vi "MPExxx_Auto_Seq_example.vi"() -> ()   [LabVIEW 2012]
doc: "This VI form enables the user to program the memory locations for auto sequencing mode and to intiate the auto sequencing mode.."
panel:
  out "error out":errorcluster
  in  "error in (no error)":errorcluster
  in  "?":enum32{"Sets Values", "Initiates Sequence"}(tab)
  in  "Memory Location":u8
  in  "Period":dbl format="%.2f"
  in  "OCP":dbl format="%.2f"
  in  "OVP":dbl format="%.2f"
  in  "Current":dbl format="%.2f"
  in  "Voltage":dbl format="%.2f"
  in  "Arm for Sequence":bool
  in  "Start":bool
  in  "VISA Resource Name":refnum<visa-resource-name>
  # "MAGNA-POWER"
  # "Electronics"
  # "Set Values for each memory location."
  # "ON"
  # "ON"
  # "OFF"
  # "OFF"
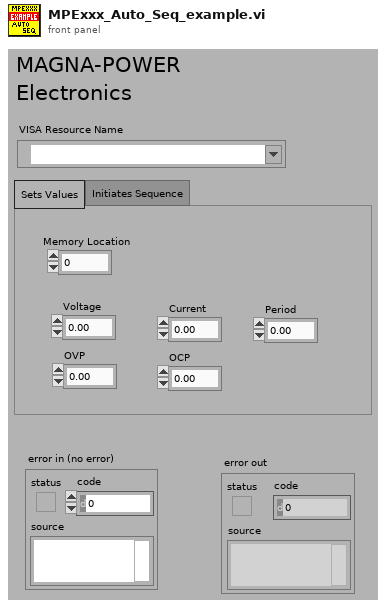
[diagram p1: front panel]
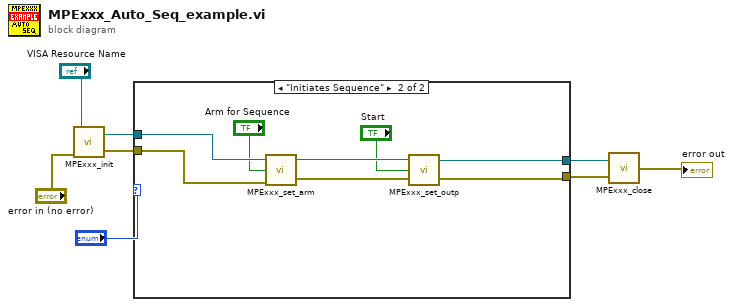
[diagram p0: block diagram]
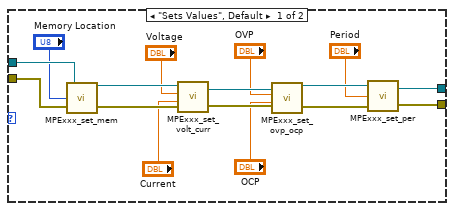
[diagram p2: hidden frame]
diagram:
  n1 = call "MPExxx_init.vi"("error in (no error)"="error in (no error)", "VISA session"="VISA Resource Name") -> ("error out"=w5:errorcluster, "dup VISA session"=w6:refnum<visa-resource-name>)  [unwired: 2 in]
  n2 = case shown="\"Initiates Sequence\"" "?" {
    tunnel: w6 -> [w24 w31]
    tunnel: w5 -> [w23 w32]
    tunnel: [w16 w27] -> w3
    tunnel: [w15 w28] -> w4
    frame "Sets Values", Default {
      n3 = call "MPExxx_set_mem.vi"("error in (no error)"=w23, "Set Mem"="Memory Location", "VISA session"=w24) -> ("error out"=w22:errorcluster, "dup VISA session"=w21:refnum<visa-resource-name>)
      n4 = call "MPExxx_set_volt_curr.vi"("error in (no error)"=w22, "Set Current"="Current", "Set Voltage"="Voltage", "VISA session"=w21) -> ("error out"=w20:errorcluster, "dup VISA session"=w19:refnum<visa-resource-name>)
      n5 = call "MPExxx_set_ovp_ocp.vi"("error in (no error)"=w20, "Set OCP"="OCP", "Set OVP"="OVP", "VISA session"=w19) -> ("error out"=w18:errorcluster, "dup VISA session"=w17:refnum<visa-resource-name>)
      n6 = call "MPExxx_set_per.vi"("error in (no error)"=w18, "Set Period"="Period", "VISA session"=w17) -> ("error out"=w15:errorcluster, "dup VISA session"=w16:refnum<visa-resource-name>)
    }
    frame "Initiates Sequence" {
      n7 = call "MPExxx_set_arm.vi"("error in (no error)"=w32, "ARM"="Arm for Sequence", "VISA session"=w31) -> ("error out"=w30:errorcluster, "dup VISA session"=w29:refnum<visa-resource-name>)
      n8 = call "MPExxx_set_outp.vi"("error in (no error)"=w30, "Output Control"="Start", "VISA session"=w29) -> ("error out"=w28:errorcluster, "dup VISA session"=w27:refnum<visa-resource-name>)
    }
  }
  n9 = call "MPExxx_close.vi"("error in (no error)"=w4, "VISA session"=w3) -> ("error out"=→"error out":errorcluster)
